vi "Write slave diagnostics.vi"(8 "error in":errorcluster, 10 "slave diagnostics":T1[](array[typedef]), 11 "Profibus Module configuration in":refnum<class "Profibus Module configuration.lvclass">) -> (0 "error out":errorcluster, 3 "Profibus Module configuration out":refnum<class "Profibus Module configuration.lvclass">)   [LabVIEW 2013, in "Profibus Module configuration.lvclass"]
uses:
  Profibus Module configuration.lvclass
  slave diagnostic configuration.ctl
  <vilib>/NI/Tag Bus Module Framework/channel/TBM channel.lvclass
  error throw specification.ctl
  Profibus Module configuration.lvclass/Profibus Module configuration.ctl
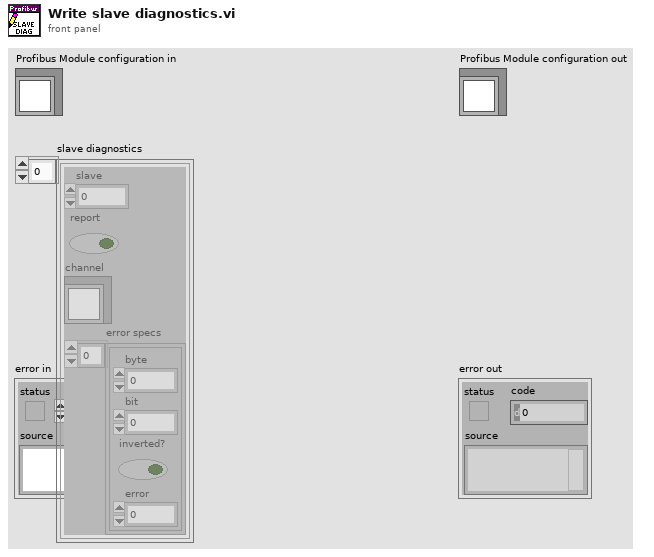
[diagram p1: front panel]
types:
  T1 = typedef "Profibus Module configuration.lvclass/slave diagnostic configuration.ctl" = cluster{"slave":i8, "report":bool, "channel":refnum<class "TBM channel.lvclass">, "error specs":T2[]}
  T2 = typedef "Profibus Module configuration.lvclass/error throw specification.ctl" = cluster{"byte":i32, "bit":i32, "inverted?":bool, "error":i32}
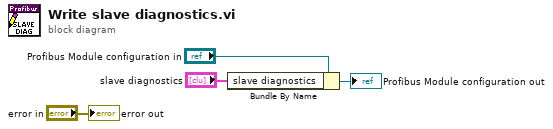
[diagram p0: block diagram]
diagram:
  n1 = Bundle By Name(cluster="Profibus Module configuration in", "slave diagnostics"="slave diagnostics") -> (→"Profibus Module configuration out":refnum<class "Profibus Module configuration.lvclass">)
  "error out" <- "error in"
